vi "Add Position.vi"(11 "named_position":T1) -> (0 "error out":errorcluster, 3 "named_positions":T1[](array[typedef]))   [LabVIEW 2020, in "Manipulator.lvlib"]
uses:
  Manipulator.lvlib
  Named Position.ctl
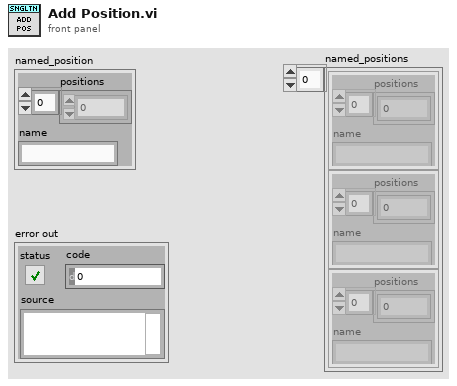
[diagram p1: front panel]
types:
  T1 = typedef "Manipulator.lvlib/Named Position.ctl" = cluster{"positions":dbl[], "name":string}
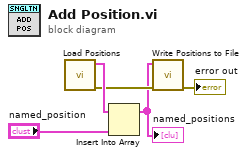
[diagram p0: block diagram]
diagram:
  n1 = call "Load Positions.vi"() -> ("error out"=w3:errorcluster, "positions"=w5:T1[])  [unwired: 10 in]
  n2 = Insert Into Array(array=w5, new element="named_position") -> (w1:T1[])  [unwired: 1 in]
  "named_positions" <- w1
  n3 = call "Write Positions to File.vi"("error in (no error)"=w3, "positions"=w1) -> ("error out"=→"error out":errorcluster)  [unwired: 9 in]
